vi "Clear Radix Core.vi"(8 "error in":errorcluster, 11 "GObjects":refnum<vi>[](array[refnum])) -> (2 "Successful":bool)   [LabVIEW 2019]
doc: "Recursively removes the Radix and Display Format from all controls and constants ."
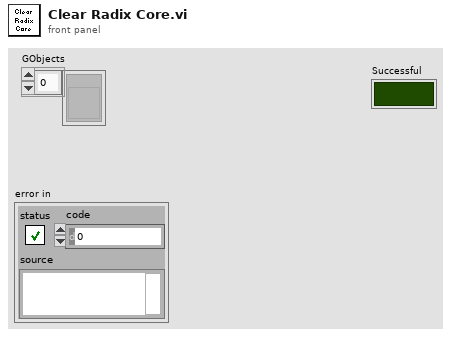
[diagram p1: front panel]
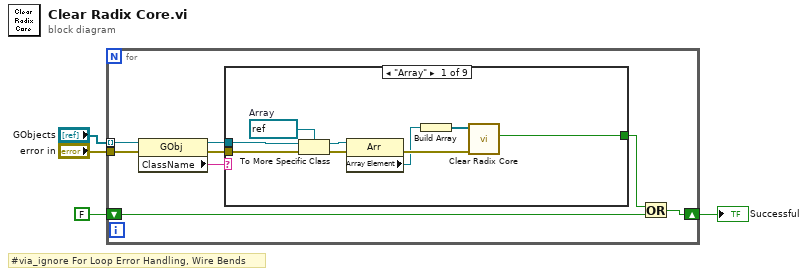
[diagram p0: block diagram]
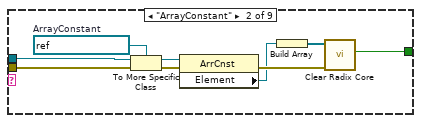
[diagram p2: hidden frame]
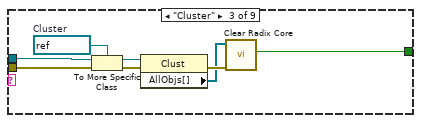
[diagram p3: hidden frame]
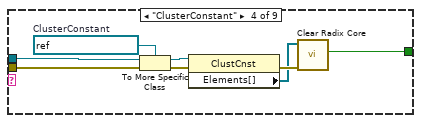
[diagram p4: hidden frame]
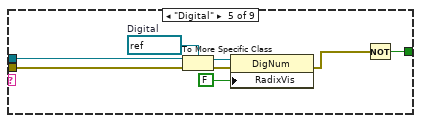
[diagram p5: hidden frame]
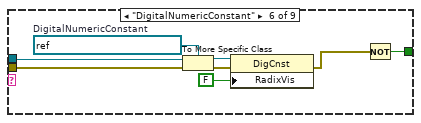
[diagram p6: hidden frame]
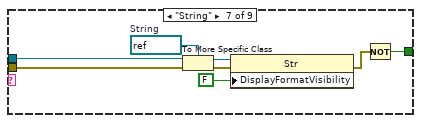
[diagram p7: hidden frame]
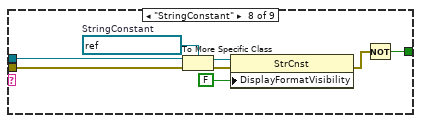
[diagram p8: hidden frame]
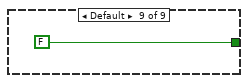
[diagram p9: hidden frame]
diagram:
  # "#via_ignore For Loop Error Handling, Wire Bends"
  n1 = for {
    shift-right: [w9] -> w2
    shift-left: FALSE -> [w10]
    tunnel: "GObjects" -> [w8] mode=indexing
    tunnel: "error in" -> [w12]
    n2 = property on="Property Node" class="GObj"(reference=w8, error in=w12) -> (reference out=w7:refnum<vi>, error out=w11:errorcluster, "ClassName"=w5:string)
    n3 = case shown="\"Array\"" w5 {
      tunnel: w11 -> [w21 w30 w37 w45 w53 w60 w68 w76 _]
      tunnel: w7 -> [w17 w26 w34 w42 w50 w55 w64 w71 _]
      tunnel: [w13 w24 w31 w39 w47 w56 w63 w72 FALSE] -> w6
      frame "Array" {
        w18 = refnum<vi> refnum  # Array
        n4 = To More Specific Class(target class=w18, reference=w17, error in=w21) -> (specific class reference=w16:refnum<vi>, error out=w20:errorcluster)
        n5 = property on="Property Node" class="Arr"(reference=w16, error in=w20) -> (error out=w19:errorcluster, "Array Element"=w15:refnum<vi>)  [unwired: 1 out]
        n6 = Build Array(w15) -> (w14:refnum<vi>[])
        n7 = call "Clear Radix Core.vi"("error in"=w19, "GObjects"=w14) -> ("Successful"=w13:bool)  [unwired: 9 in]
      }
      frame "ArrayConstant" {
        w27 = refnum<vi> refnum  # ArrayConstant
        n8 = To More Specific Class(target class=w27, reference=w26, error in=w30) -> (specific class reference=w25:refnum<vi>, error out=w29:errorcluster)
        n9 = property on="Property Node" class="ArrCnst"(reference=w25, error in=w29) -> (error out=w28:errorcluster, "Element"=w23:refnum<vi>)  [unwired: 1 out]
        n10 = Build Array(w23) -> (w22:refnum<vi>[])
        n11 = call "Clear Radix Core.vi"("error in"=w28, "GObjects"=w22) -> ("Successful"=w24:bool)  [unwired: 9 in]
      }
      frame "Cluster" {
        w35 = refnum<vi> refnum  # Cluster
        n12 = To More Specific Class(target class=w35, reference=w34, error in=w37) -> (specific class reference=w33:refnum<vi>, error out=w38:errorcluster)
        n13 = property on="Property Node" class="Clust"(reference=w33, error in=w38) -> (error out=w36:errorcluster, "AllObjs[]"=w32:refnum<vi>[])  [unwired: 1 out]
        n14 = call "Clear Radix Core.vi"("error in"=w36, "GObjects"=w32) -> ("Successful"=w31:bool)  [unwired: 9 in]
      }
      frame "ClusterConstant" {
        w43 = refnum<vi> refnum  # ClusterConstant
        n15 = To More Specific Class(target class=w43, reference=w42, error in=w45) -> (specific class reference=w41:refnum<vi>, error out=w46:errorcluster)
        n16 = property on="Property Node" class="ClustCnst"(reference=w41, error in=w46) -> (error out=w44:errorcluster, "Elements[]"=w40:refnum<vi>[])  [unwired: 1 out]
        n17 = call "Clear Radix Core.vi"("error in"=w44, "GObjects"=w40) -> ("Successful"=w39:bool)  [unwired: 9 in]
      }
      frame "Digital" {
        w51 = refnum<vi> refnum  # Digital
        n18 = To More Specific Class(target class=w51, reference=w50, error in=w53) -> (specific class reference=w49:refnum<vi>, error out=w54:errorcluster)
        n19 = property on="Property Node" class="DigNum"(reference=w49, error in=w54, "RadixVis"=FALSE ("Radix Visible?")) -> (error out=w52:errorcluster)  [unwired: 1 out]
        n20 = Not(x=w52) -> (.not. x?=w47:bool)
      }
      frame "DigitalNumericConstant" {
        w59 = refnum<vi> refnum  # DigitalNumericConstant
        n21 = To More Specific Class(target class=w59, reference=w55, error in=w60) -> (specific class reference=w58:refnum<vi>, error out=w62:errorcluster)
        n22 = property on="Property Node" class="DigCnst"(reference=w58, error in=w62, "RadixVis"=FALSE ("Radix Visible?")) -> (error out=w61:errorcluster)  [unwired: 1 out]
        n23 = Not(x=w61) -> (.not. x?=w56:bool)
      }
      frame "String" {
        w67 = refnum<vi> refnum  # String
        n24 = To More Specific Class(target class=w67, reference=w64, error in=w68) -> (specific class reference=w66:refnum<vi>, error out=w70:errorcluster)
        n25 = property on="Property Node" class="Str"(reference=w66, error in=w70, "DisplayFormatVisibility"=FALSE ("Radix Visible?")) -> (error out=w69:errorcluster)  [unwired: 1 out]
        n26 = Not(x=w69) -> (.not. x?=w63:bool)
      }
      frame "StringConstant" {
        w75 = refnum<vi> refnum  # StringConstant
        n27 = To More Specific Class(target class=w75, reference=w71, error in=w76) -> (specific class reference=w74:refnum<vi>, error out=w78:errorcluster)
        n28 = property on="Property Node" class="StrCnst"(reference=w74, error in=w78, "DisplayFormatVisibility"=FALSE ("Radix Visible?")) -> (error out=w77:errorcluster)  [unwired: 1 out]
        n29 = Not(x=w77) -> (.not. x?=w72:bool)
      }
      frame Default {
      }
    }
    n30 = Or(x=w6, y=w10) -> (x .or. y?=w9:bool)
  }
  "Successful" <- w2
